vi "LWXPS_PositionerAnalogTrackingPositionParametersGet.vi"(0 "XPS Reference IN":refnum<k24>, 7 "Positioner Name":string, 11 "LabVIEW error IN":errorcluster) -> (2 "XPS Reference OUT":refnum<k24>, 3 "Returned error code":i32, 4 "Analog Input Name":string, 6 "Offset":dbl, 8 "Scale":dbl, 10 "Velocity":dbl, 13 "LabVIEW error OUT":errorcluster, 14 "XPS Error String":string, 15 "Acceleration":dbl)   [LabVIEW 2014]
uses:
  D:/XPSQ8_LabView_Library/Development/Source/Dll/Newport.XPS.CommandInterface.dll
  Dll/Newport.XPS.CommandInterface.dll
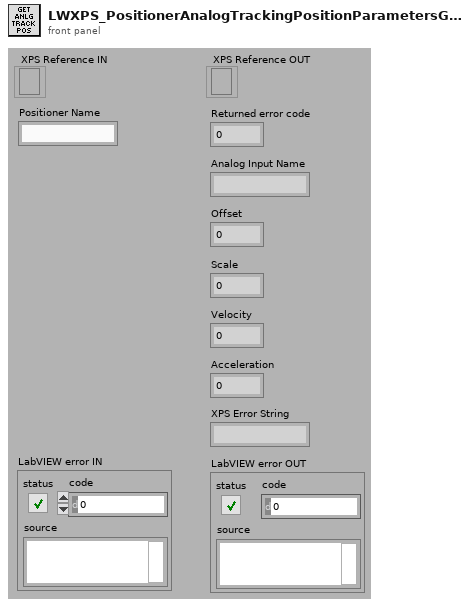
[diagram p1: front panel]
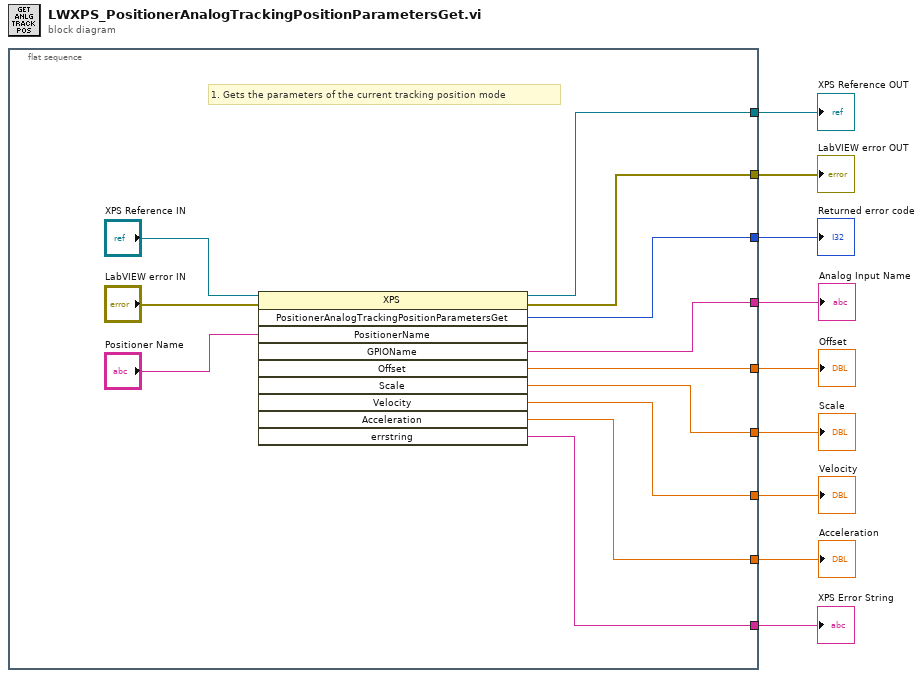
[diagram p0: block diagram]
diagram:
  n1 = flat-sequence {
    tunnel: [w15] -> w5
    tunnel: [w20] -> w9
    tunnel: [w19] -> w8
    tunnel: [w18] -> w7
    tunnel: [w14] -> w4
    tunnel: [w13] -> w3
    tunnel: [w12] -> w2
    tunnel: [w11] -> w1
    tunnel: [w10] -> w6
    frame #0 {
      # "1. Gets the parameters of the current tracking position mode"
      n2 = invoke class="XPS" method="PositionerAnalogTrackingPositionParametersGet"(reference="XPS Reference IN", error in="LabVIEW error IN", "PositionerName"="Positioner Name") -> (reference out=w20:refnum<k24>, error out=w19:errorcluster, "PositionerAnalogTrackingPositionParametersGet"=w18:i32, "GPIOName"=w15:string, "Offset"=w14:dbl, "Scale"=w13:dbl, "Velocity"=w12:dbl, "Acceleration"=w11:dbl, "errstring"=w10:string)  [unwired: 7 in, 1 out]
    }
  }
  "XPS Error String" <- w6
  "XPS Reference OUT" <- w9
  "LabVIEW error OUT" <- w8
  "Returned error code" <- w7
  "Analog Input Name" <- w5
  "Offset" <- w4
  "Scale" <- w3
  "Velocity" <- w2
  "Acceleration" <- w1
